vi "CRYUpdate Project Control State.vi"(10 "VI Ref":refnum<vi>, 11 "RefTree In":refnum<vi>) -> (2 "State FlgArray":bool[](array[boolean]), 3 "RefTree Out":refnum<vi>)   [LabVIEW 2013]
uses:
  CRYProject Editor Global.vi
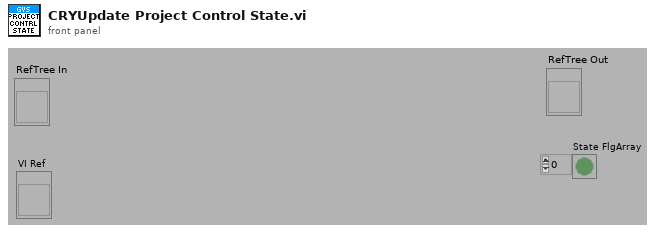
[diagram p1: front panel]
types:
  T1 = typedef "CRYTS.ctl" = cluster{"No.TS":u16, "TS File Path":path, "TS Name":string, "EditStepName":string, "Steps":T2[], "New State":bool, "Change State":bool, "Flattened CurveLib Data":string, "Document Data":string, "EditStepNo":u16, "Operator Start File":string, "Sequence Type":string, "Sequence Language":string}
  T2 = typedef "CRYStep.ctl" = cluster{"No.VI":i32, "Category":string, "StepName":string, "Seq setup flattened":string, "Comment":string, "Steps config.":bool[], "Jump config":i32[], "Start":dbl, "Increment":dbl, "Name":string, "Unit":string, "Y data":u16, "Y prefix":string, "Y dB ref":dbl, "Y unit":string, "Repeat State Array":cluster{"Start":dbl, "Increment":dbl, "Count":i32, "Num":i32}[]}
  T3 = enum8{"Enabled", "Disabled", "Disabled and Grayed Out"}
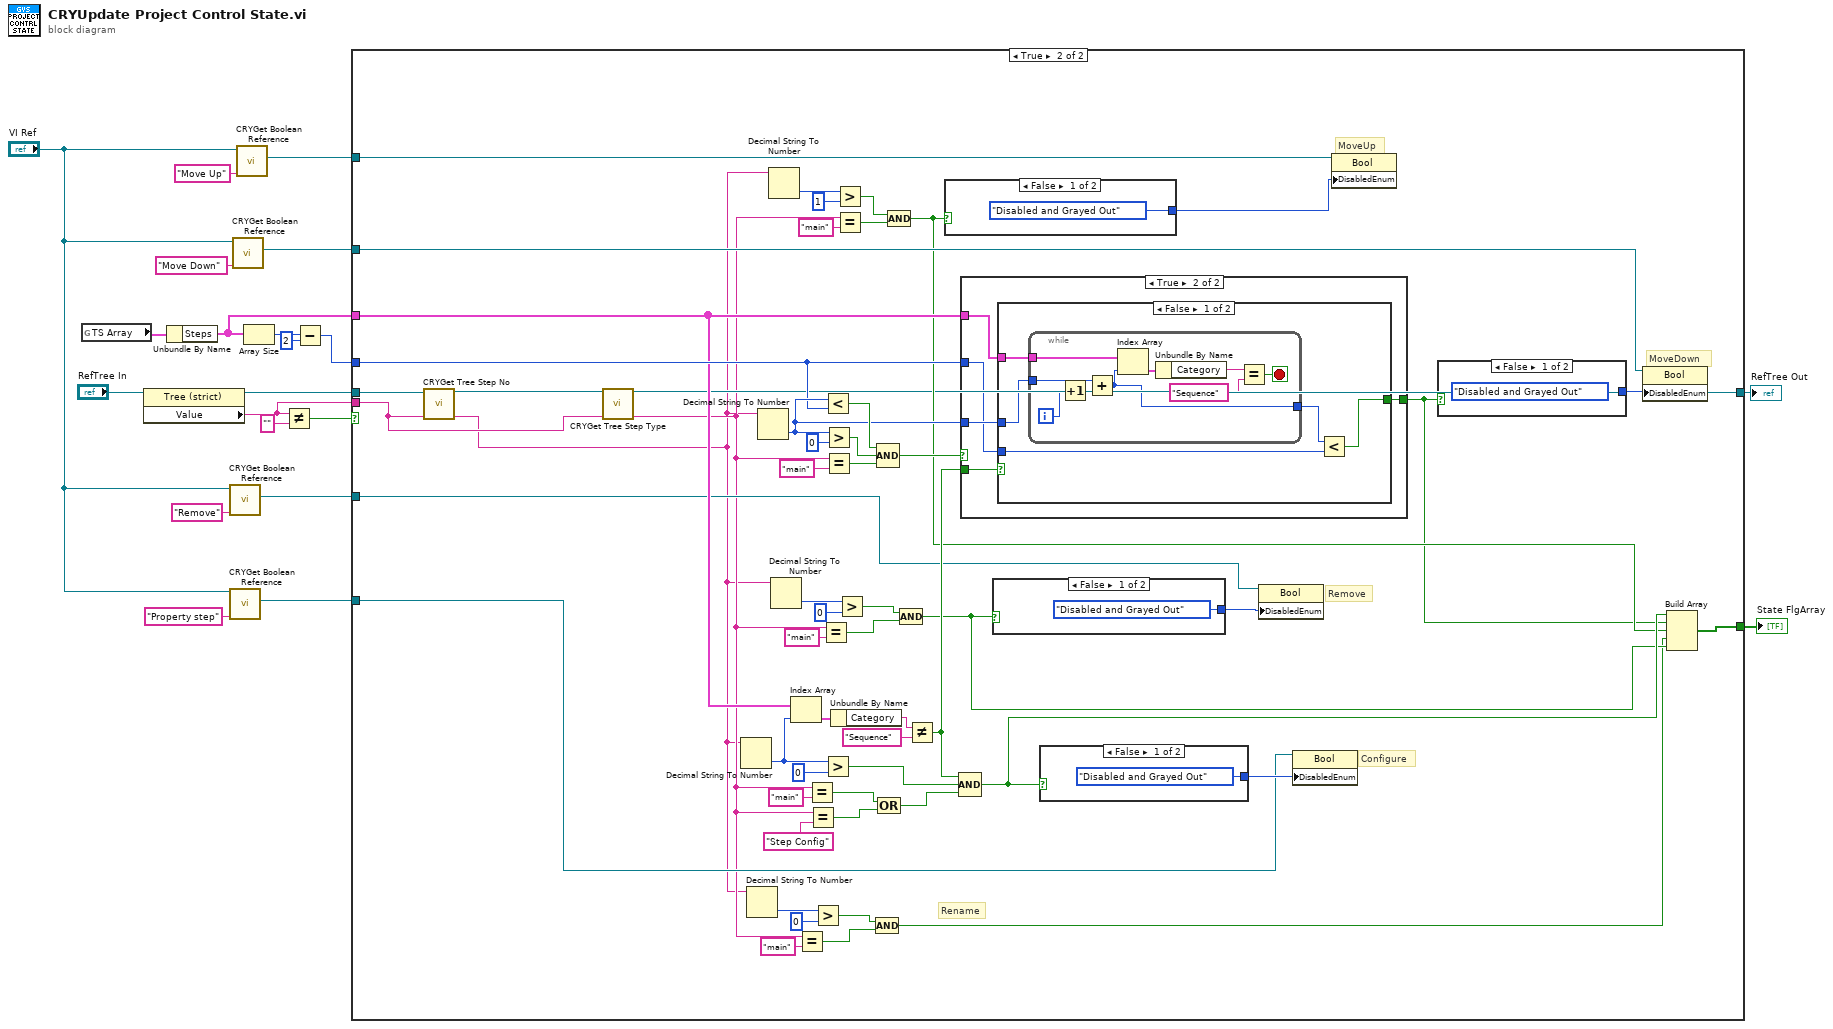
[diagram p0: block diagram]
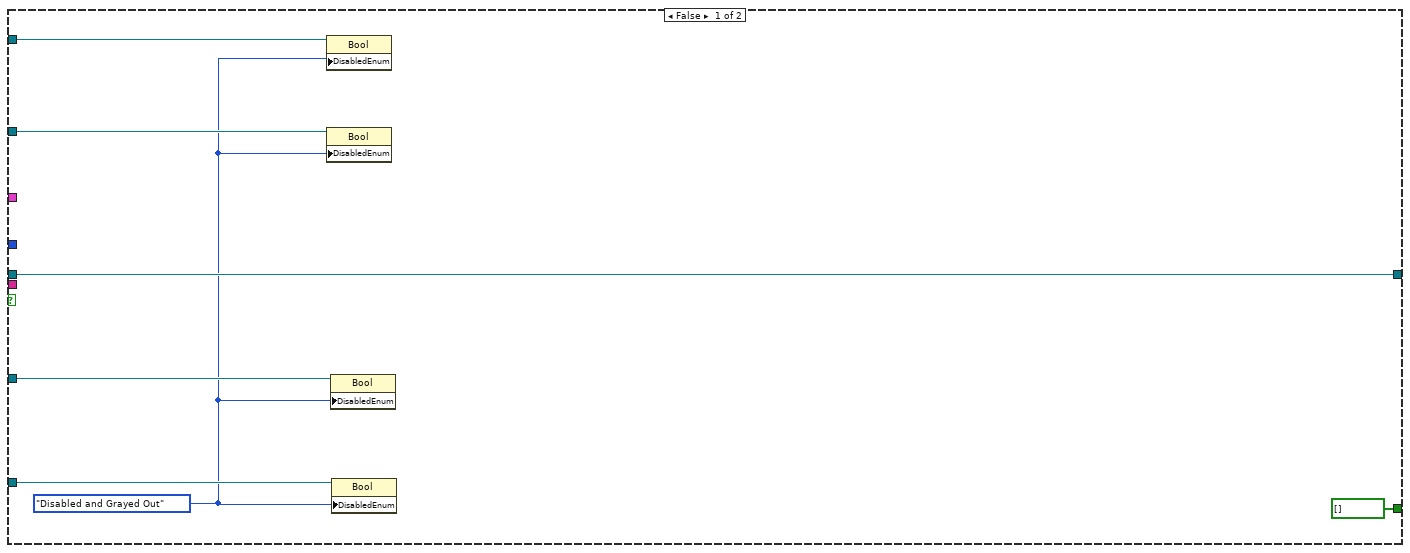
[diagram p2: hidden frame]
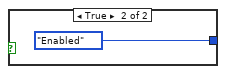
[diagram p3: hidden frame]
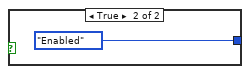
[diagram p4: hidden frame]
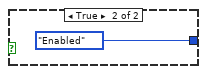
[diagram p5: hidden frame]
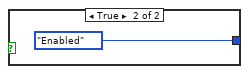
[diagram p6: hidden frame]
diagram:
  n1 = global read "CRYProject Editor Global.vi" "TS Array"() -> (w17:T1)
  n2 = property on="Property Node" class="Tree (strict)"(reference="RefTree In") -> (reference out=w12:refnum<vi>, "Value"=w11:string)  [unwired: 1 in, 1 out]
  n3 = Unbundle By Name(w17) -> ("Steps"=w16:T2[])
  n4 = call "CRYGet Boolean Reference.vi"("Label Name"="Remove", "VI Refnum"="VI Ref") -> ("Boolean Ref"=w5:refnum<vi>)  [unwired: 9 out]
  n5 = call "CRYGet Boolean Reference.vi"("Label Name"="Property step", "VI Refnum"="VI Ref") -> ("Boolean Ref"=w4:refnum<vi>)  [unwired: 9 out]
  n6 = call "CRYGet Boolean Reference.vi"("Label Name"="Move Down", "VI Refnum"="VI Ref") -> ("Boolean Ref"=w6:refnum<vi>)  [unwired: 9 out]
  n7 = call "CRYGet Boolean Reference.vi"("Label Name"="Move Up", "VI Refnum"="VI Ref") -> ("Boolean Ref"=w7:refnum<vi>)  [unwired: 9 out]
  n8 = Array Size(array=w16) -> (size(s)=w10:i32)
  n9 = Not Equal?(x=w11, y="") -> (x != y?=w13:bool)
  n10 = Subtract(x=w10, y=2) -> (x-y=w8:i32)
  n11 = case shown="True" w13 {
    tunnel: w12 -> [w28 w45]
    tunnel: w11 -> [_ w43]
    tunnel: w8 -> [_ w79]
    tunnel: w16 -> [_ w63]
    tunnel: w7 -> [w27 w61]
    tunnel: w6 -> [w26 w59]
    tunnel: w5 -> [w25 w57]
    tunnel: w4 -> [w24 w55]
    tunnel: [w28 w42] -> w3
    tunnel: [bool[] [] w53] -> w1
    frame False {
      w23 = T3."Disabled and Grayed Out" ("Disabled")
      n12 = property class="Bool"(reference=w27, "DisabledEnum"=w23) -> ()  [unwired: 1 in, 2 out]
      n13 = property class="Bool"(reference=w26, "DisabledEnum"=w23) -> ()  [unwired: 1 in, 2 out]
      n14 = property class="Bool"(reference=w25, "DisabledEnum"=w23) -> ()  [unwired: 1 in, 2 out]
      n15 = property class="Bool"(reference=w24, "DisabledEnum"=w23) -> ()  [unwired: 1 in, 2 out]
    }
    frame True {
      # "Rename"
      # "MoveUp"
      # "MoveDown"
      # "Remove"
      # "Configure"
      n16 = call "CRYGet Tree Step No.vi"("SequenceTree"=w45, "Active Item Tag"=w43) -> ("reference out"=w44:refnum<vi>, "Active Cell String4"=w31:string)  [unwired: 12 in]
      n17 = call "CRYGet Tree Step Type.vi"("SequenceTree"=w44, "Active Item Tag"=w43) -> ("reference out"=w42:refnum<vi>, "Active Cell String3"=w32:string)  [unwired: 12 in]
      n18 = Decimal String To Number(string=w31) -> (number=w70:i32)  [unwired: 2 in, 1 out]
      n19 = Decimal String To Number(string=w31) -> (number=w33:i32)  [unwired: 2 in, 1 out]
      n20 = Decimal String To Number(string=w31) -> (number=w80:i32)  [unwired: 2 in, 1 out]
      n21 = Decimal String To Number(string=w31) -> (number=w77:i32)  [unwired: 2 in, 1 out]
      n22 = Decimal String To Number(string=w31) -> (number=w74:i32)  [unwired: 2 in, 1 out]
      n23 = Index Array(array=w63, index=w70) -> (element=w71:T2)
      n24 = Equal?(x=w32, y="main" ("decimal integer string")) -> (x = y?=w36:bool)
      n25 = Equal?(x=w32, y="main" ("decimal integer string")) -> (x = y?=w40:bool)
      n26 = Equal?(x=w32, y="Step Config" ("SequenceName")) -> (x = y?=w39:bool)
      n27 = Greater?(x=w33, y=0) -> (0:w35:bool)
      n28 = Equal?(x=w32, y="main" ("decimal integer string")) -> (x = y?=w65:bool)
      n29 = Less?(x=w80, y=w79) -> (x < y?=w81:bool)
      n30 = Greater?(x=w70, y=0) -> (0:w67:bool)
      n31 = Greater?(x=w80, y=0) -> (0:w83:bool)
      n32 = Equal?(x=w32, y="main" ("decimal integer string")) -> (x = y?=w84:bool)
      n33 = Unbundle By Name(w71) -> ("Category"=w69:string)
      n34 = Greater?(x=w77, y=1) -> (0:w75:bool)
      n35 = Equal?(x=w32, y="main" ("decimal integer string")) -> (x = y?=w78:bool)
      n36 = Greater?(x=w74, y=0) -> (0:w66:bool)
      n37 = Compound Arithmetic op=AND(w35, w36) -> (w29:bool)
      n38 = Compound Arithmetic op=AND(w81, w83, w84) -> (w52:bool)
      n39 = Compound Arithmetic op=OR(w40, w39) -> (w38:bool)
      n40 = Compound Arithmetic op=AND(w75, w78) -> (w51:bool)
      n41 = Compound Arithmetic op=AND(w66, w65) -> (w30:bool)
      n42 = Not Equal?(x=w69, y="Sequence" ("Category")) -> (x != y?=w64:bool)
      n43 = case shown="False" w51 {
        tunnel: [T3."Disabled and Grayed Out" ("Disabled") T3."Enabled" ("Disabled")] -> w62
        frame False {
        }
        frame True {
        }
      }
      n44 = Compound Arithmetic op=AND(w64, w67, w38) -> (w54:bool)
      n45 = case shown="True" w52 {
        selector: w52 -> [w93 _]
        tunnel: [w93 w98] -> w50
        tunnel: w63 -> [_ w97]
        tunnel: w80 -> [_ w96]
        tunnel: w79 -> [_ w95]
        tunnel: w64 -> [_ w94]
        frame False {
        }
        frame True {
          n46 = case shown="False" w94 {
            selector: w94 -> [_ w113]
            tunnel: [w99 w113] -> w98
            tunnel: w97 -> [w103 _]
            tunnel: w96 -> [w102 _]
            tunnel: w95 -> [w100 _]
            frame False {
              n47 = while {
                tunnel: w103 -> [w112]
                tunnel: w102 -> [w111]
                tunnel: [w104] -> w101
                i -> [w105]
                stop <- w106 stop-if-true
                n48 = Increment(x=w105) -> (x+1=w110:i32)
                n49 = Add(x=w111, y=w110) -> (x+y=w104:i32)
                n50 = Index Array(array=w112, index=w104) -> (element=w109:T2)
                n51 = Unbundle By Name(w109) -> ("Category"=w108:string)
                n52 = Equal?(x=w108, y="Sequence") -> (x = y?=w106:bool)
              }
              n53 = Less?(x=w101, y=w100) -> (x < y?=w99:bool)
            }
            frame True {
            }
          }
        }
      }
      n54 = case shown="False" w30 {
        tunnel: [T3."Disabled and Grayed Out" ("Disabled") T3."Enabled" ("Disabled")] -> w58
        frame False {
        }
        frame True {
        }
      }
      n55 = case shown="False" w54 {
        tunnel: [T3."Disabled and Grayed Out" ("Disabled") T3."Enabled" ("Disabled")] -> w56
        frame False {
        }
        frame True {
        }
      }
      n56 = property class="Bool"(reference=w57, "DisabledEnum"=w58) -> ()  [unwired: 1 in, 2 out]
      n57 = property on="Property Node" class="Bool"(reference=w55, "DisabledEnum"=w56) -> ()  [unwired: 1 in, 2 out]
      n58 = property class="Bool"(reference=w61, "DisabledEnum"=w62) -> ()  [unwired: 1 in, 2 out]
      n59 = case shown="False" w50 {
        tunnel: [T3."Disabled and Grayed Out" ("Disabled") T3."Enabled" ("Disabled")] -> w60
        frame False {
        }
        frame True {
        }
      }
      n60 = property class="Bool"(reference=w59, "DisabledEnum"=w60) -> ()  [unwired: 1 in, 2 out]
      n61 = Build Array(w54, w50, w51, w29, w30) -> (w53:bool[])
    }
  }
  "RefTree Out" <- w3
  "State FlgArray" <- w1
